vi "Init Interface.vi"(8 "error in":errorcluster, 9 "Config Section":string, 10 "hse-config":refnum<class "config-base.lvclass">, 11 "DB-ADO":refnum<class "DB-ADO.lvclass">) -> (0 "error out":errorcluster, 3 "DB-ADO":refnum<class "DB-ADO.lvclass">)   [LabVIEW 2020, in "hse-db-ado.lvlib" / "DB-ADO.lvclass"]
doc: "____\nHAMPEL SOFTWARE ENGINEERING v1.4.0 (2023-12-19 09:52)"
uses:
  DB-ADO.lvclass
  hse-libraries/Source/hse-configuration/config-base/config-base.lvclass
  hse-libraries/Source/hse-application/hse-application.lvclass/hse-application.ctl
  hse-libraries/Source/hse-application/HSE Application not initialized--error.vi
  <vilib>/Utility/error.llb/Clear Errors.vi
  hse-libraries/Source/hse-application/hse-application__GetSingleton.vi
  <vilib>/Utility/sysdir.llb/Get System Directory.vi
  <vilib>/Utility/error.llb/Error Cluster From Error Code.vi
  DB-ADO.lvclass/DB-ADO.ctl
  hse-libraries/Source/hse-application/hse-application.lvclass
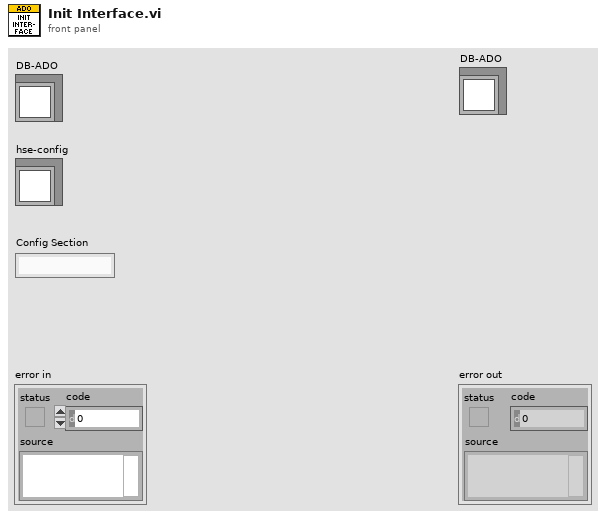
[diagram p1: front panel]
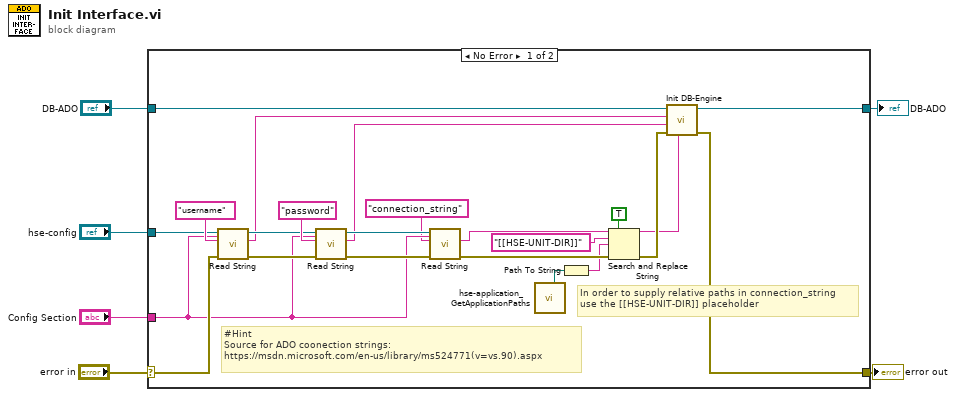
[diagram p0: block diagram]
diagram:
  n1 = case shown="No Error" "error in" {
    selector: "error in" -> [w29 w31]
    tunnel: [w28 w31] -> w5
    tunnel: [w26 w30] -> w1
    tunnel: "DB-ADO" -> [w27 w30]
    tunnel: "hse-config" -> [w19 _]
    tunnel: "Config Section" -> [w18 _]
    frame No Error {
      # "In order to supply relative paths in connection_string\nuse the [[HSE-UNIT-DIR]] placeholder"
      # "#Hint\nSource for ADO coonection strings:\nhttps://msdn.microsoft.com/en-us/library/ms524771(v=vs.90).aspx"
      n2 = call-dynamic "Read String.vi"("Section"=w18, "error in"=w29, "Key"="username", "config-base in"=w19) -> ("error out"=w20:errorcluster, "Value"=w17:string, "config-base out"=w21:refnum<class "config-base.lvclass">)  [unwired: 5 in]
      n3 = call-dynamic "Read String.vi"("Section"=w18, "error in"=w20, "Key"="password", "config-base in"=w21) -> ("error out"=w24:errorcluster, "Value"=w16:string, "config-base out"=w25:refnum<class "config-base.lvclass">)  [unwired: 5 in]
      n4 = call-dynamic "Read String.vi"("Section"=w18, "error in"=w24, "Key"="connection_string", "config-base in"=w25) -> ("error out"=w11:errorcluster, "Value"=w8:string)  [unwired: 5 in, 1 out]
      n5 = call "hse-application_GetApplicationPaths.vi"() -> ("Config/Unit Directory"=w14:path)  [unwired: 5 in, 6 out]
      n6 = Path To String(path=w14) -> (string=w7:string)
      n7 = Search and Replace String(replace all?=TRUE ("replace all? (F)"), input string=w8, search string="[[HSE-UNIT-DIR]]" ("Key"), replace string=w7, error in=w11) -> (result string=w9:string, error out=w10:errorcluster)  [unwired: 3 in, 2 out]
      n8 = call-dynamic "Init DB-Engine.vi"("Database"=w9, "error in"=w10, "Password"=w16, "User"=w17, "DB-Engine in"=w27) -> ("error out"=w28:errorcluster, "DB-Engine out"=w26:refnum<class "DB-ADO.lvclass">)  [unwired: 5 in]
    }
    frame Error {
    }
  }
  "error out" <- w5
  "DB-ADO" <- w1
